vi "7L18-c-Couts_optimum.vi"(5 "error in":errorcluster caption="err in", 9 "Pièce":T1) -> (0 "Coût (q=Qe)":T2, 3 "Pièce Maj":T1, 4 "error out":errorcluster caption="err out")   [LabVIEW 2010, in "lv_07.lvlib"]
doc: "Optimum économique (Qe - Te -CSM)\nSi T<0 alors T initialisé à 0,15\nSi Cc<0 alors Cc initialisé à 20 euros\nPièce Maj est modifié avec les valeurs initialisées le cas échéant"
uses:
  lv_07.lvlib
  c_cout_choix_q.ctl
  c_pi_wilson.ctl
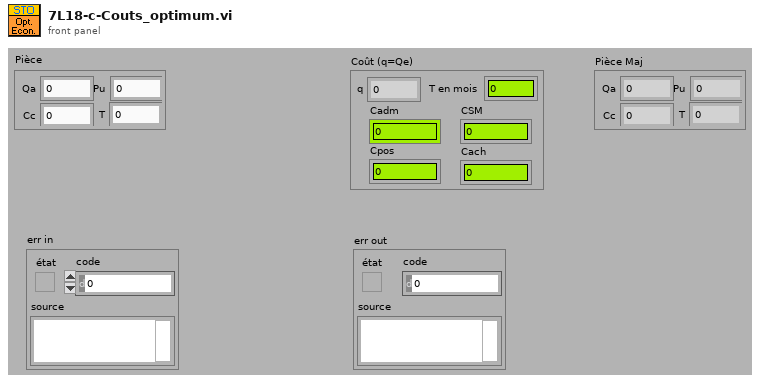
[diagram p1: front panel]
types:
  T1 = typedef "lv_07.lvlib/c_pi_wilson.ctl" = cluster{"T":dbl, "Pu":dbl, "Qa":dbl, "Cc":dbl}
  T2 = typedef "lv_07.lvlib/c_cout_choix_q.ctl" = cluster{"Cadm":dbl, "Cpos":dbl, "Cach":dbl, "CSM":dbl, "q":dbl, "T en mois":dbl}
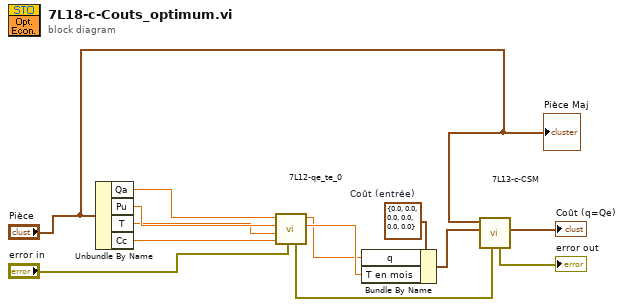
[diagram p0: block diagram]
diagram:
  w6 = T2 {"Cadm"=0.0, "Cpos"=0.0, "Cach"=0.0, "CSM"=0.0, "q"=0.0, "T en mois"=0.0}  # Coût (entrée)
  n1 = Unbundle By Name("Pièce") -> ("Qa"=w7:dbl, "Pu"=w8:dbl, "T"=w2:dbl, "Cc"=w1:dbl)
  n2 = call "7L12-qe_te_0.vi"("err in"="error in", "Cc"=w1, "T"=w2, "Pu"=w8, "Qa"=w7) -> ("Te (en mois)"=w10:dbl, "Qe"=w9:dbl, "error out"=w4:errorcluster)  [unwired: 4 in]
  n3 = Bundle By Name(cluster=w6, "q"=w9, "T en mois"=w10) -> (w11:T2)
  n4 = call "7L13-c-CSM.vi"("err in"=w4, "Coût (e)"=w11, "Pièce (e)"="Pièce") -> ("Coût (s)"=→"Coût (q=Qe)":T2, "err out"=→"error out":errorcluster)  [unwired: 5 in]
  "Pièce Maj" <- "Pièce"
